vi "Configure Deguass and Offset Rate.vi"(8 "error in (no error)":errorcluster, 10 "Deguass and Offset Rate ( 1 )":i32=1, 11 "VISA resource name":refnum<visa-resource-name>) -> (0 "error out":errorcluster, 3 "VISA resource out":refnum<visa-resource-name>)   [LabVIEW 2011, in "Ocean Server OS4000.lvlib"]
doc: "Set the frequency at which the sensor should degauss and offset operations.\n\nThe quicker you degauss the lower the compass lag is when moving it quickly."
uses:
  Ocean Server OS4000.lvlib
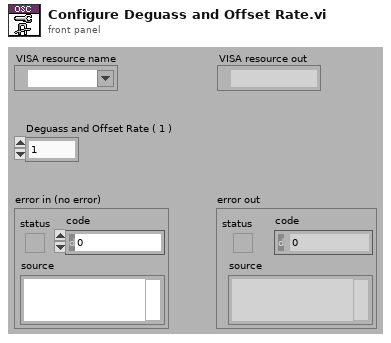
[diagram p1: front panel]
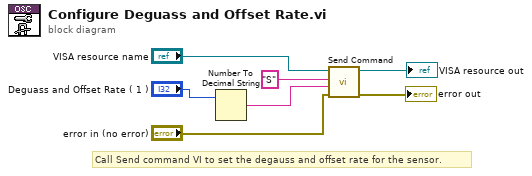
[diagram p0: block diagram]
diagram:
  # "Call Send command VI to set the degauss and offset rate for the sensor."
  n1 = Number To Decimal String(number="Deguass and Offset Rate ( 1 )") -> (decimal integer string=w4:string)  [unwired: 1 in]
  n2 = call "Send Command.vi"("error in (no error)"="error in (no error)", "Value"=w4, "Message"="S", "VISA resource name"="VISA resource name") -> ("error out"=→"error out":errorcluster, "VISA resource out"=→"VISA resource out":refnum<visa-resource-name>)  [unwired: 6 in]
